vi "EK-P4 Global.vi"() -> ()   [LabVIEW 2016]
doc: "global for event references. To have less inputs and outpus to the various VIs. Only main writes to the global, at the beginning. everyone else only reads."
panel:
  in  "Stop User Event":refnum<user-event>
  in  "Start User Event":refnum<user-event>
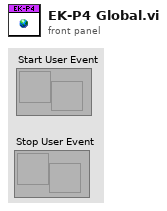
[diagram p1: front panel]
diagram:
